vi "while loop sevo control temp.vi"() -> ()   [LabVIEW 2022 SP3]
uses:
  <vilib>/DAQmx/create/channels.llb/DAQmx Create Channel (DO-Digital Output).vi
panel:
  in  "Slide":dbl(slide) scale=1.0..2.0
  in  "stop":bool
  in  "lines 2":tag
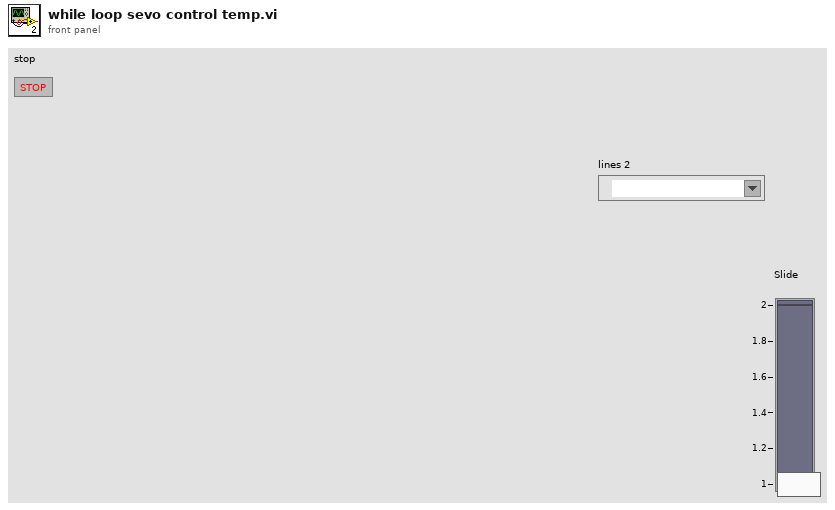
[diagram p1: front panel]
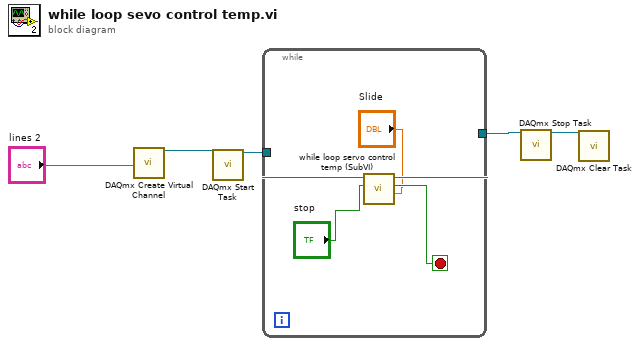
[diagram p0: block diagram]
diagram:
  n1 = call-poly <vilib>:"DAQmx Create Virtual Channel.vi"("lines"="lines 2") -> ("task out"=w4:refnum<k21>)  [unwired: 13 in, 1 out]
  n2 = call <vilib>:"DAQmx Start Task.vi"("task/channels in"=w4) -> ("task out"=w3:refnum<k21>)  [unwired: 13 in, 1 out]
  n3 = while {
    tunnel: w3 -> [w10]
    tunnel: [w7] -> w1
    stop <- w8 stop-if-true
    n4 = call "while loop servo control temp (SubVI).vi"("Slide"="Slide", "stop in"="stop", "Refnum in"=w10) -> ("stop out"=w8:bool, "Refnum out"=w7:refnum<k21>)  [unwired: 7 in]
  }
  n5 = call <vilib>:"DAQmx Stop Task.vi"("task/channels in"=w1) -> ("task out"=w2:refnum<k21>)  [unwired: 13 in, 1 out]
  n6 = call <vilib>:"DAQmx Clear Task.vi"("task in"=w2) -> ()  [unwired: 14 in, 1 out]
